vi "readNumberOfImagesXML.vi"(8 "error in (no error)":errorcluster, 10 "NativeXML in":refnum<class "NativeXML.lvclass">, 11 "PixelflySettings in":refnum<class "PixelflySettings.lvclass">) -> (0 "error out":errorcluster, 2 "NativeXML out":refnum<class "NativeXML.lvclass">, 3 "PixelflySettings out":refnum<class "PixelflySettings.lvclass">)   [LabVIEW 2011, in "Tools.lvlib" / "Settings.lvlib" / "PixelflySettings.lvclass"]
uses:
  PixelflySettings.lvclass
  NativeXML/NativeXML.lvclass
  PixelflySettings.lvclass/PixelflySettings.ctl
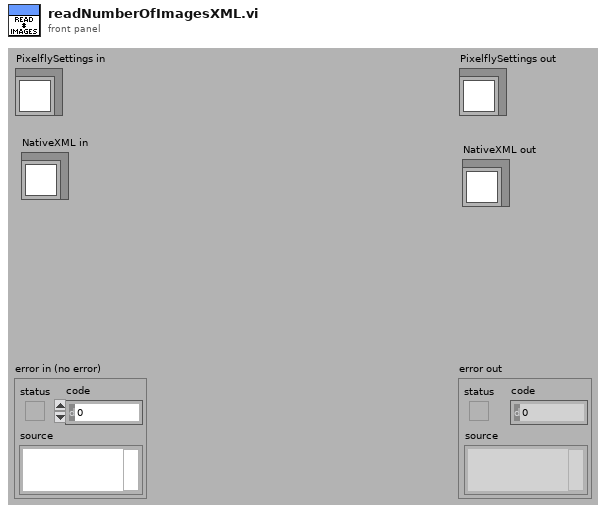
[diagram p1: front panel]
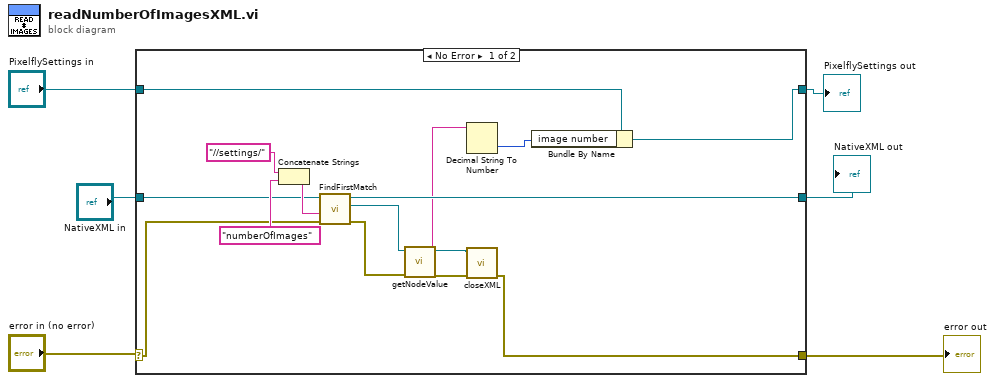
[diagram p0: block diagram]
diagram:
  n1 = case shown="No Error" "error in (no error)" {
    selector: "error in (no error)" -> [w11 w22]
    tunnel: [w17 w22] -> w5
    tunnel: [w20 w23] -> w4
    tunnel: "PixelflySettings in" -> [w21 w23]
    tunnel: "NativeXML in" -> [w9 w24]
    tunnel: [w14 w24] -> w1
    frame No Error {
      n2 = Concatenate Strings("//settings/" ("searchElementIn"), "numberOfImages") -> (w10:string)
      n3 = call "FindFirstMatch.vi"("error in (no error)"=w11, "xPath"=w10, "NativeXML in"=w9) -> ("error out"=w12:errorcluster, "NativeXML match"=w13:refnum<class "NativeXML.lvclass">, "NativeXML out"=w14:refnum<class "NativeXML.lvclass">)  [unwired: 6 in]
      n4 = call "getNodeValue.vi"("error in (no error)"=w12, "NativeXML in"=w13) -> ("error out"=w18:errorcluster, "Value"=w7:string, "NativeXML out"=w19:refnum<class "NativeXML.lvclass">)  [unwired: 7 in]
      n5 = Decimal String To Number(string=w7) -> (number=w8:i32)  [unwired: 2 in, 1 out]
      n6 = call "closeXML.vi"("error in (no error)"=w18, "NativeXML in"=w19) -> ("error out"=w17:errorcluster)  [unwired: 9 in]
      n7 = Bundle By Name(cluster=w21, "image number"=w8) -> (w20:refnum<class "PixelflySettings.lvclass">)
    }
    frame Error {
    }
  }
  "error out" <- w5
  "PixelflySettings out" <- w4
  "NativeXML out" <- w1
